vi "ReadLightColor.vi"(4 "error in (no error)":errorcluster, 6 "Container State":T3, 7 "Display State In":T1) -> (0 "error out":errorcluster, 2 "Value":u32(colorbox), 3 "Display State Out":T1)   [LabVIEW 2013, in "BarCodes.lvlib" / "Barcode.xctl"]
uses:
  Barcode.xctl
  <vilib>/_xctls/Container State.ctl
  State.ctl
  BarcodeType.ctl
  <vilib>/_xctls/XControlSupport.lvlib
  BarCodes.lvlib
panel:
  # "Replace the Value Indicator below with an Indicator of desired type.\nDo not remove this Indicator or the others from the connector pane. \nDo not change the connector pane pattern.\nThe Value Indicator should always be the second terminal from top on the output side in the connector pane."
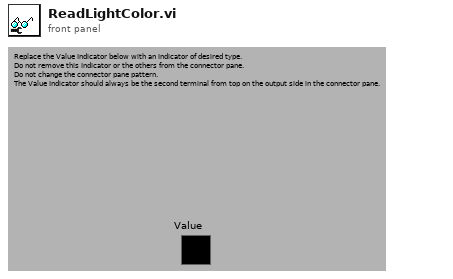
[diagram p1: front panel]
types:
  T1 = typedef "BarCodes.lvlib/Barcode.xctl/State.ctl" = cluster{"BarcodeType":T2, "Scale":u8, "Dark Color":u32, "Light Color":u32}
  T2 = typedef "BarCodes.lvlib/BarcodeType.ctl" = enum16{"EAN-13", "UPC", "Code 39 (3 of 9)", "Code 128"}
  T3 = typedef "XControlSupport.lvlib/Container State.ctl" = cluster{"Indicator?":bool, "Run Mode?":bool, " Refnum":refnum<vi>}
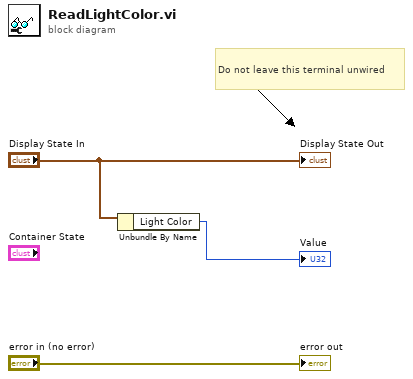
[diagram p0: block diagram]
diagram:
  # "Do not leave this terminal unwired"
  n1 = Unbundle By Name("Display State In") -> ("Light Color"=→"Value":u32)
  "error out" <- "error in (no error)"
  "Display State Out" <- "Display State In"
